vi "Read Timer.vi"(8 "error in (no error)":errorcluster, 11 "Channel GUI in":refnum<class "Channel GUI.lvclass">) -> (0 "error out":errorcluster, 2 "Timer":u32, 3 "Channel GUI out":refnum<class "Channel GUI.lvclass">)   [LabVIEW 2018, in "Channel GUI.lvclass"]
uses:
  Channel GUI.lvclass
  Channel GUI.lvclass/Channel GUI.ctl
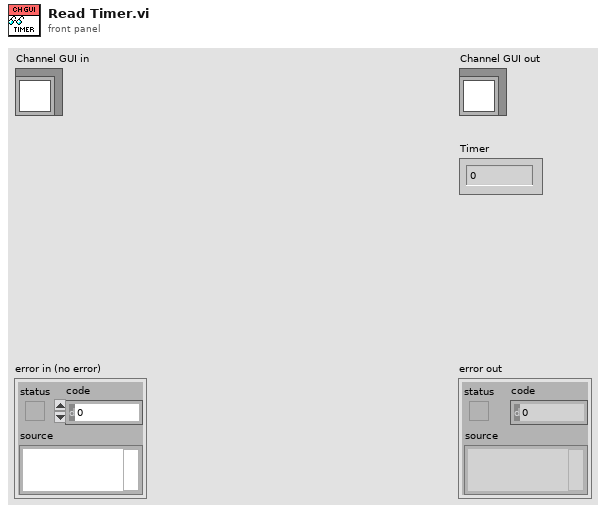
[diagram p1: front panel]
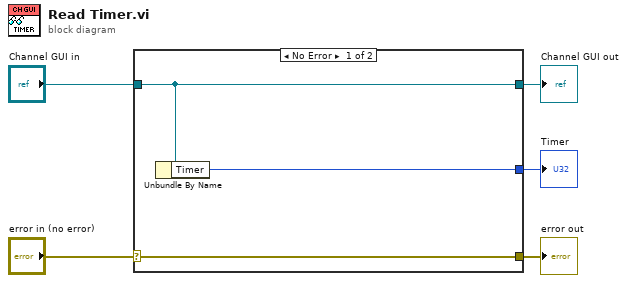
[diagram p0: block diagram]
diagram:
  n1 = case shown="No Error" "error in (no error)" {
    selector: "error in (no error)" -> [w8 w9]
    tunnel: [w8 w9] -> w4
    tunnel: [w7 w10] -> w2
    tunnel: "Channel GUI in" -> [w7 w10]
    tunnel: [w6 _] -> w1
    frame No Error {
      n2 = Unbundle By Name(w7) -> ("Timer"=w6:u32)
    }
    frame Error {
    }
  }
  "error out" <- w4
  "Channel GUI out" <- w2
  "Timer" <- w1
